vi "Lockin API State Machine.vi"() -> ()   [LabVIEW 2019]
uses:
  Instrument.Lockin/Instrument.Lockin.lvclass
  <userlib>/_OpenG.lib/error/error.llb/openg_error.lvlib
  <userlib>/_OpenG.lib/error/error.llb/Filter Error Codes (Array)__ogtk.vi
  Instrument.Lockin/Typedefs/API/Lockin.Commands--Enum.ctl
  Instrument.Lockin/Typedefs/Results Type--Enum.ctl
  Instrument.DAQ/Typedefs/AO.Channel.Function--Enum.ctl
  Instrument.DAQ/Instrument.DAQ.lvclass
  Instrument.DAQ/Typedefs/AO.Channel--Cluster.ctl
  Instrument.DAQ/Typedefs/AO.Channel--Cluster--Array.ctl
  Instrument.DAQ/Typedefs/REF.Channel--Cluster.ctl
  Instrument.DAQ/Typedefs/REF.Channel--Cluster--Array.ctl
panel:
  in  "Tab Control":T1(tab)=enum."config"
  out "getResults":dbl[](graph)
  in  "Type":T2
  out "getAO":waveform(dbl)[](graph)
  out "getAI":waveform(dbl)[](graph)
  in  "Reset":bool
  in  "Channels: AO":T3 {"Phase" format="%#_3g"; "Frequency" min=0.0001 max=200000.0 format="%#_6p"; "Offset" format="%#_6p"; "Amplitude" min=0.0 max=10.0 format="%#_6p"}
  in  "Channels: Lockin in":T6=[{"Enable?"=FALSE, "Channel"=13, "Frequency"=0.1, "Phase"=0.0, "TC"=1e-05, "Roll-Off"=1}] {"Roll-Off" min=1; "TC" min=0.0001 format="%#_3p"; "Phase" format="%#_3g"; "Frequency" min=0.0001 max=200000.0 format="%#_6p"; "Channel" min=1}
  in  "Trigger":bool
  out "timeout (ms)":u32=202
  in  "side gate channel":i32=1
  in  "phase":dbl
  in  "cycles (1,2,...)":i32=1 min=1 step=1
  in  "Vmin (start)":dbl=-0.15 format="%#_3p"
  in  "Vmax (end)":dbl=0.7 format="%#_3p"
  in  "dV":dbl=0.0005 format="%#_3p"
  in  "function (ramp)":enum16{"Ramp", "Triangle", "Sine"}(ring)
  out "getResults 2":cluster{"Waveform Graph":dbl[], dbl[]}(graph)
  in  "address":string
  in  "Enum":T8
  in  "Stop":bool
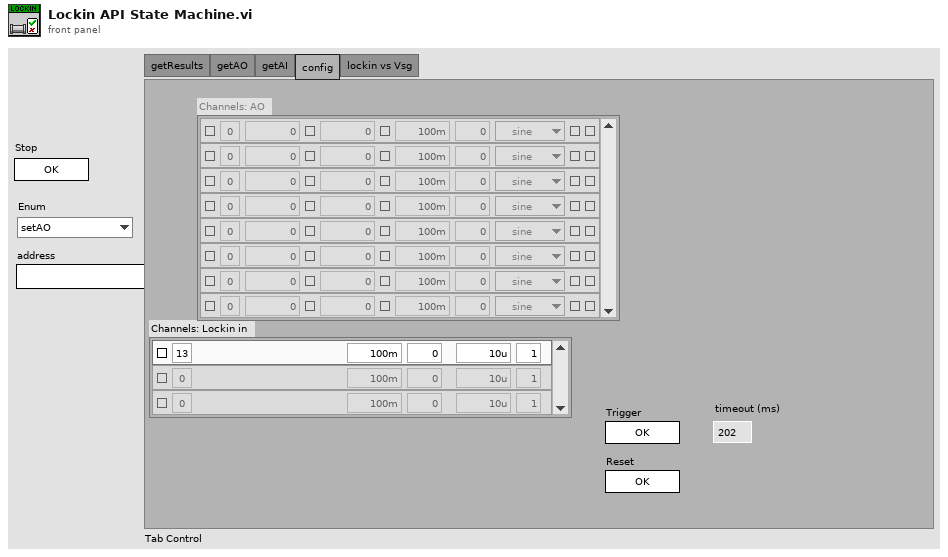
[diagram p1: front panel]
types:
  T1 = enum32{"getResults", "getAO", "getAI", "config", "lockin vs Vsg"}
  T2 = typedef "Instrument.Lockin.lvlib/Instrument.Lockin.lvclass/Results Type--Enum.ctl" = enum16{"X", "Y", "R", "Theta", "Mean"}
  T3 = typedef "Instrument.Lockin.lvlib/Instrument.DAQ.lvclass/AO.Channel--Cluster--Array.ctl" = T4[]
  T4 = typedef "Instrument.Lockin.lvlib/Instrument.DAQ.lvclass/AO.Channel--Cluster.ctl" = cluster{"Enable?":bool, "Channel":i32, "Amplitude":dbl, "Offset":dbl, "Frequency":dbl, "Phase":dbl, "Function":T5, "Sweeping?":bool, "Limit AC":bool, "Limit DC?":bool, "Duty Cycle":bool}
  T5 = typedef "Instrument.Lockin.lvlib/Instrument.DAQ.lvclass/AO.Channel.Function--Enum.ctl" = enum16{"sine", "square", "triangle", "saw"}
  T6 = typedef "Instrument.Lockin.lvlib/Instrument.DAQ.lvclass/REF.Channel--Cluster--Array.ctl" = T7[]
  T7 = typedef "Instrument.Lockin.lvlib/Instrument.DAQ.lvclass/REF.Channel--Cluster.ctl" = cluster{"Enable?":bool, "Channel":i32, "Frequency":dbl, "Phase":dbl, "TC":dbl, "Roll-Off":i32}
  T8 = typedef "Instrument.Lockin.lvlib/Instrument.Lockin.lvclass/Lockin.Commands--Enum.ctl" = enum16{"setAO", "setAO_Amplitude", "setAO_DC", "setAO_Frequency", "setAO_Phase", "setAO_Function", "setREF", "setREF_Frequency", "setREF_Phase", "setREF_TC", "setREF_Roll-Off", "setDAQ", "setSampling", "setState", "getState", "getAO", "getAI", "getResults", "getSampling", "getAOconfig", "getREFconfig", "setInputGain", "setOutputGain", "getInputGain", "getOutputGain", "setSamplingFsMode", "getSamplingFsMode", "setSweep", "setSweep_Time", "setSweep_Table", "getStatus", "getSweepResults", "getSweepWaveforms", "logConfiguration", "startLogging", "stopLogging"}
  T9 = enum32{"invalid app kind", "Development System", "Run Time System", "Student Edition", "Embedded LabVIEW", "Evaluation", "Custom"}
  T10 = enum32{"Invalid", "Standard", "Closed", "Hidden", "Minimized", "Maximized"}
  T11 = cluster{"Core":cluster{"Current VI Reference":refnum<vi>, "Close Panel on Exit?":bool}, "Lockin":refnum<class "Instrument.Lockin.lvclass">}
  T12 = cluster{"Current VI Reference":refnum<vi>, "Close Panel on Exit?":bool}
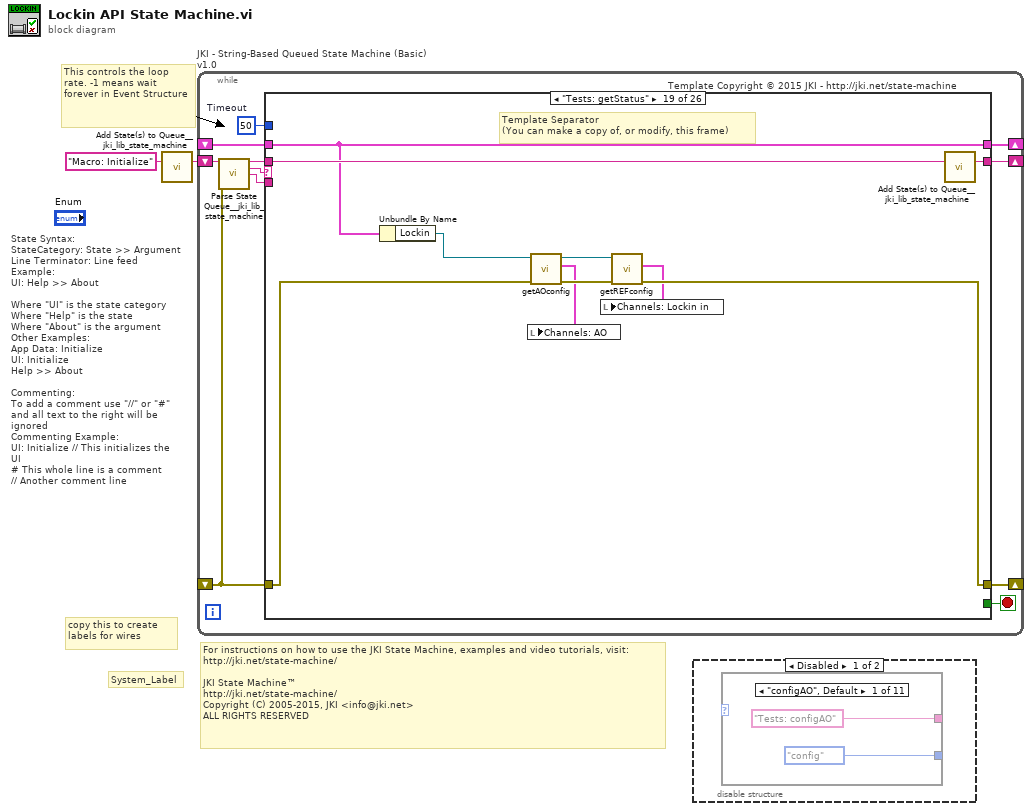
[diagram p0: block diagram]
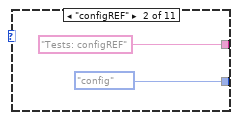
[diagram p2: hidden frame]
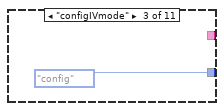
[diagram p3: hidden frame]
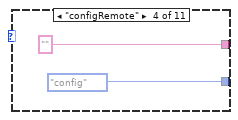
[diagram p4: hidden frame]
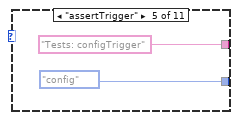
[diagram p5: hidden frame]
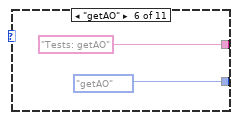
[diagram p6: hidden frame]
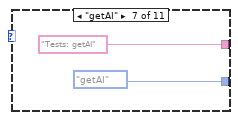
[diagram p7: hidden frame]
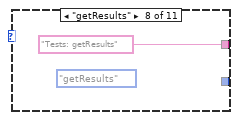
[diagram p8: hidden frame]
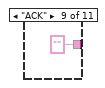
[diagram p9: hidden frame]
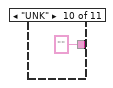
[diagram p10: hidden frame]
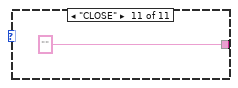
[diagram p11: hidden frame]
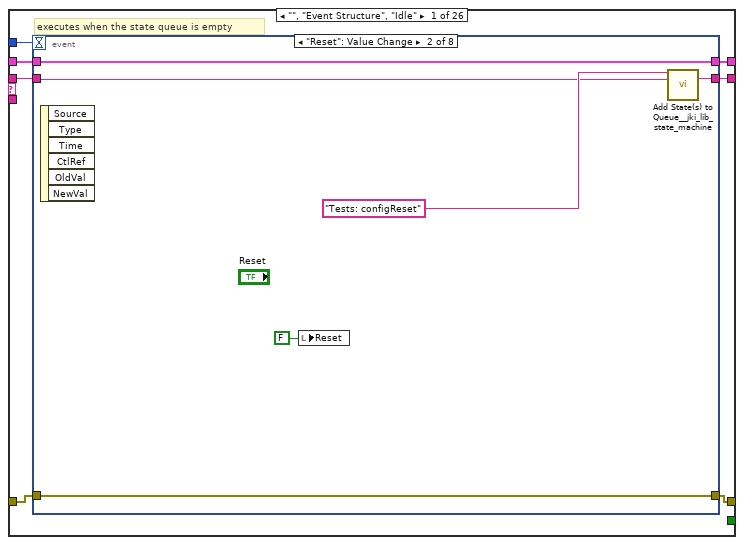
[diagram p13: hidden frame]
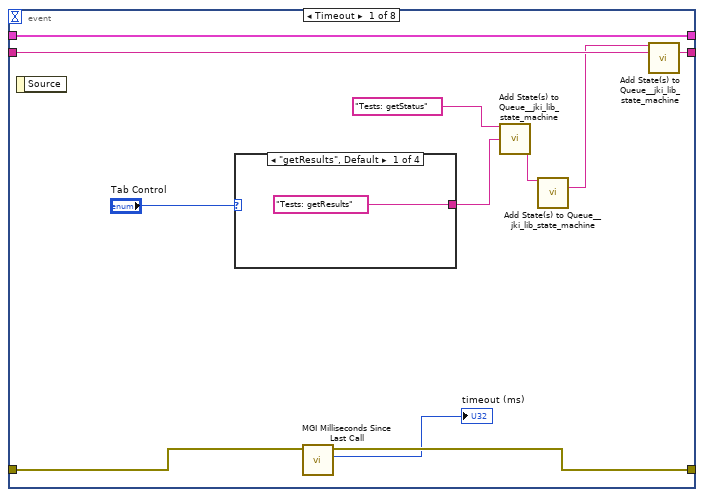
[diagram p14: hidden frame]
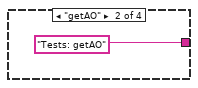
[diagram p15: hidden frame]
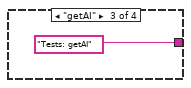
[diagram p16: hidden frame]
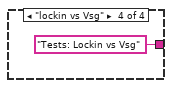
[diagram p17: hidden frame]
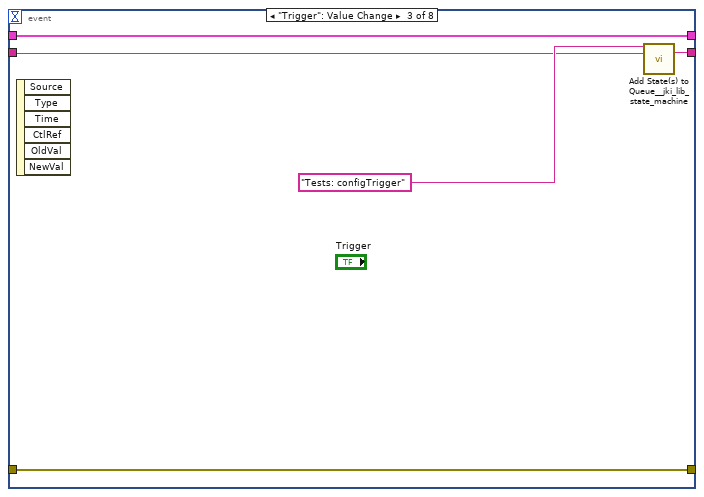
[diagram p18: hidden frame]
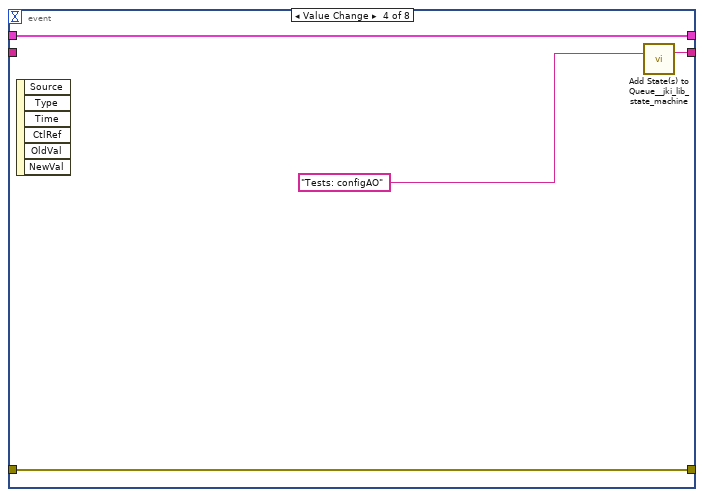
[diagram p19: hidden frame]
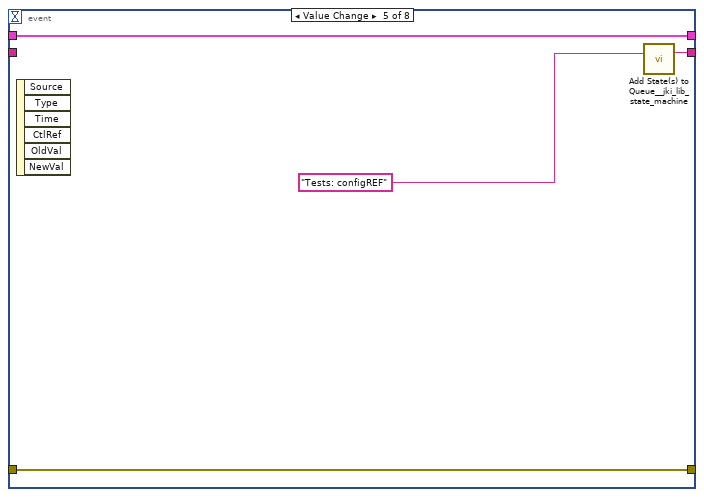
[diagram p20: hidden frame]
diagram:
  # "For instructions on how to use the JKI State Machine, examples and video tutorials, visit:\nhttp://jki.net/state-machine/\n\nJKI State Machine™\nhttp://jki.net/state-machine/\nCopyright (C) 2005-2015, JKI <info@jki.net>\nALL RIGHTS RESERVED"
  # "State Syntax:\nStateCategory: State >> Argument\nLine Terminator: Line feed\nExample:\nUI: Help >> About\n\nWhere \"UI\" is the state category\nWhere \"Help\" is the state\nWhere \"About\" is the argument\nOther Examples:\nApp Data: Initialize\nUI: Initialize\nHelp >> About\n\nCommenting:\nTo add a comment use \"//\" or \"#\" and all text to the right will be ignored\nCommenting Example:\nUI: Initialize // This initializes the UI\n# This whole line is a comment\n// Another comment line"
  # "copy this to create labels for wires"
  # "This controls the loop rate. -1 means wait forever in Event Structure"
  # "System_Label"
  n1 = call <vilib>:"Add State(s) to Queue__jki_lib_state_machine.vi"("State(s) in (\"\")"="Macro: Initialize") -> ("States Out"=w2:string)  [unwired: 14 in]
  n2 = while "JKI - String-Based Queued State Machine (Basic) v1.0" {
    shift-right: [w6] -> _
    shift-left: _ -> [w5]
    shift-right: [w9] -> _
    shift-left: _ -> [w3]
    shift-right: [w8] -> _
    shift-left: w2 -> [w10]
    stop <- w7 stop-if-true
    w4 = 50  # Timeout
    # "Template Copyright © 2015 JKI - http://jki.net/state-machine"
    n3 = call <vilib>:"Parse State Queue__jki_lib_state_machine.vi"("State Queue"=w10, "Error In (no error)"=w3) -> ("Remaining States"=w12:string, "Current State"=w13:string, "Arguments"=w11:string)  [unwired: 11 in]
    n4 = case shown="\"Tests: getStatus\"" w13 {
      selector: w13 -> [_ _ w79 _ _ _ _ _ _ _ _ _ _ _ _ _ _ _ _ _ _ _ _ _ _ _]
      tunnel: w12 -> [w20 w78 w83 w101 w109 w114 w118 w124 w130 w134 w138 w144 w155 w181 w186 w196 w200 w210 w220 w227 w234 w241 w248 w254 w260 w277]
      tunnel: w11 -> [_ _ _ _ _ _ _ _ _ _ _ w139 w149 _ _ _ _ _ _ _ _ _ _ _ _ _]
      tunnel: w5 -> [w18 w75 w81 w92 w106 w112 w115 _ w125 w131 w136 w142 w151 w178 w183 w193 w197 w207 w218 w223 w230 w237 w244 w252 w257 w265]
      tunnel: [w17 w76 w85 w98 errorcluster {"status"=FALSE, "code"=0, "source"=""} ("error out") w111 w116 w121 w126 w132 w135 w140 w152 w179 w184 w194 w198 w201 w215 w224 w231 w238 w245 w250 w256 w275] -> w9
      tunnel: w3 -> [w16 w76 w84 w98 w104 w111 w116 w121 w127 w132 w135 w141 w153 w179 w184 w194 w198 w208 w216 w225 w232 w239 w246 w251 w258 w275]
      tunnel: [w19 w77 w82 w100 w108 w113 w117 w123 w129 w133 w137 w143 w154 w180 w185 w195 w199 w209 w219 w226 w233 w240 w247 w253 w259 w276] -> w8
      tunnel: [_ _ _ _ _ TRUE _ _ _ _ _ _ _ _ _ _ _ _ _ _ _ _ _ _ _ _] -> w7
      tunnel: [w15 w75 w81 w99 w106 w112 w115 w122 w125 w131 w136 w142 w151 w178 w183 w193 w197 w207 w218 w223 w230 w237 w244 w252 w257 w265] -> w6
      tunnel: w4 -> [w14 _ _ _ _ _ _ _ _ _ _ _ _ _ _ _ _ _ _ _ _ _ _ _ _ _]
      frame "", "Event Structure", "Idle" {
        # "executes when the state queue is empty"
        n5 = event shown="[1] \"Reset\": Value Change" {
          selector: _ -> [_ _ _ _ _ _ _ _]
          dyn-events: _ -> [_ _ _ _ _ _ _ _]
          timeout: w14 -> [_ _ _ _ _ _ _ _]
          tunnel: w20 -> [w31 w37 w42 _ _ w62 w68 w74]
          tunnel: [w30 w41 w46 w50 w54 w63 w67 w73] -> w19
          tunnel: w18 -> [w29 w38 w43 w48 w52 w58 w65 w71]
          tunnel: [w22 w39 w44 w49 w53 w55 w66 w72] -> w17
          tunnel: w16 -> [w23 w39 w44 w49 w53 w56 w66 w72]
          tunnel: [w29 w38 w43 w48 w52 w61 w65 w71] -> w15
          event Timeout {
            n6 = event-data() -> ()  [unwired: 1 in, 1 out]
            n7 = case shown="\"getResults\", Default" "Tab Control" {
              tunnel: ["Tests: getResults" "Tests: getAO" "Tests: getAI" "Tests: Lockin vs Vsg"] -> w27
              frame "getResults", Default {
              }
              frame "getAO" {
              }
              frame "getAI" {
              }
              frame "lockin vs Vsg" {
              }
            }
            n8 = call <userlib>:"MGI Milliseconds Since Last Call.vi"("Error In"=w23) -> ("ms"=→"timeout (ms)":u32, "Error Out"=w22:errorcluster)  [unwired: 5 in]
            n9 = call <vilib>:"Add State(s) to Queue__jki_lib_state_machine.vi"("State(s) in Front (\"\")"="Tests: getStatus", "State(s) at Back (\"\")"=w27) -> ("States Out"=w25:string)  [unwired: 13 in]
            n10 = call <vilib>:"Add State(s) to Queue__jki_lib_state_machine.vi"("State(s) in Front (\"\")"=w25) -> ("States Out"=w24:string)  [unwired: 14 in]
            n11 = call <vilib>:"Add State(s) to Queue__jki_lib_state_machine.vi"("State(s) in Front (\"\")"=w24, "State(s) in (\"\")"=w31) -> ("States Out"=w30:string)  [unwired: 13 in]
          }
          event "Reset": Value Change {
            n12 = event-data() -> ()  [unwired: 1 in, 6 out]
            n13 = local write "Reset"(FALSE ("Reset")) -> ()
            n14 = call <vilib>:"Add State(s) to Queue__jki_lib_state_machine.vi"("State(s) in Front (\"\")"="Tests: configReset", "State(s) in (\"\")"=w37) -> ("States Out"=w41:string)  [unwired: 13 in]
          }
          event "Trigger": Value Change {
            n15 = event-data() -> ()  [unwired: 1 in, 6 out]
            n16 = call <vilib>:"Add State(s) to Queue__jki_lib_state_machine.vi"("State(s) in Front (\"\")"="Tests: configTrigger", "State(s) in (\"\")"=w42) -> ("States Out"=w46:string)  [unwired: 13 in]
          }
          event Value Change {
            n17 = event-data() -> ()  [unwired: 1 in, 6 out]
            n18 = call <vilib>:"Add State(s) to Queue__jki_lib_state_machine.vi"("State(s) in (\"\")"="Tests: configAO") -> ("States Out"=w50:string)  [unwired: 14 in]
          }
          event Value Change {
            n19 = event-data() -> ()  [unwired: 1 in, 6 out]
            n20 = call <vilib>:"Add State(s) to Queue__jki_lib_state_machine.vi"("State(s) in (\"\")"="Tests: configREF") -> ("States Out"=w54:string)  [unwired: 14 in]
          }
          event "address": Value Change {
            n21 = event-data() -> ()  [unwired: 1 in, 6 out]
            n22 = Unbundle By Name(w58) -> ("Lockin"=w57:refnum<class "Instrument.Lockin.lvclass">)
            n23 = call-dynamic "Open.vi"("error in (no error)"=w56, "address"="address", "Instrument.Lockin in"=w57) -> ("error out"=w55:errorcluster, "Instrument.Lockin out"=w59:refnum<class "Instrument.Lockin.lvclass">)  [unwired: 7 in]
            n24 = Bundle By Name(cluster=w58, "Lockin"=w59) -> (w61:T11)
            n25 = call <vilib>:"Add State(s) to Queue__jki_lib_state_machine.vi"("State(s) in (\"\")"=w62) -> ("States Out"=w63:string)  [unwired: 14 in]
          }
          event "Stop": Value Change {
            # "Exit Button Value Change (pressed) Event\n(this executes Macro: Exit to terminate the VI)"
            n26 = event-data() -> ()  [unwired: 1 in, 1 out]
            n27 = call <vilib>:"Add State(s) to Queue__jki_lib_state_machine.vi"("State(s) in Front (\"\")"="Macro: Exit", "State(s) in (\"\")"=w68) -> ("States Out"=w67:string)  [unwired: 13 in]
          }
          event Panel Close? {
            # "Discard the event because we'll close the front panel ourselves in Macro: Exit"
            # "Close Panel button (pressed) Event\n(this executes Macro: Exit to terminate the VI)"
            n28 = event-data() -> ()  [unwired: 1 in, 1 out]
            n29 = event-data("Discard?"=TRUE) -> ()  [unwired: 1 in, 1 out]
            n30 = call <vilib>:"Add State(s) to Queue__jki_lib_state_machine.vi"("State(s) in Front (\"\")"="Macro: Exit", "State(s) in (\"\")"=w74) -> ("States Out"=w73:string)  [unwired: 13 in]
          }
        }
      }
      frame "---------- Core ----------" {
        # "Do not put any code in this frame.\n(it is a separator no-op)"
        n31 = call <vilib>:"Add State(s) to Queue__jki_lib_state_machine.vi"("State(s) in (\"\")"=w78) -> ("States Out"=w77:string)  [unwired: 14 in]
      }
      frame Default {
        w88 = 42 items=["No error", "Argument error", "Memory is full", "Out of zone", "End of file", "File already open", "Generic file I/O error", "File not found", "File permission error", "Disk is full", "Duplicate path", "Too many files open", "System feature not enabled", "Resource file not found", "Cannot add resource", "Resource not found", "Image not found", "Image memory error", "Pen does not exist", "Config type invalid", "Config token not found", "Config parse error", "Config memory error", "Bad external code format", "Bad external code offset", "External code not present", "Null window", "Destroy window error", "Null menu", "Print aborted", "Bad print record", "Print driver error", "Windows error during printing", "Memory error during printing", "Print dialog error", "Generic print error", "Invalid device refnum", "Device not found", "Device parameter error", "Device unit error", "Cannot open device", "Device call aborted", "Generic error", "Cancelled by user", "Object ID too low", "Object ID too high", "Object not in heap", "Unknown heap", "Unknown object (invalid DefProc)", "Unknown object (DefProc not in table)", "Message out of range", "Invalid (null) method", "Unknown message", "Manager call not supported", "Bad address", "Network operation in progress", "Network operation timed out", "Connection is busy", "Network attribute not supported", "Network error", "Address in use", "System out of memory", "Connection aborted", "Connection refused", "Not connected", "Already connected", "Connection closed", "Initialization error (interapplication manager)", "Bad occurrence", "Wait on unbound occurrence handler", "Occurrence queue overflow", "Datalog type conflict", "Unused", "Unrecognized type (interapplication manager)", "Memory corrupt", "Failed to make temporary DLL", "Old CIN version", "Drag socket not found", "Failed to load drop-object", "Failed to register OLE object", "Failed to release OLE object", "Format specifier type mismatch", "Unknown format specifier", "Too few format specifiers", "Too many format specifiers", "Scan failed", "Newer CIN version", "Error converting to variant", "Runtime menu error", "Password tampered", "Variant attribute not found", "Incompatible variant data type", "Event data is not available", "Event Store is not present", "Occurrence is not found", "Event Queue is not created", "Event info is not available", "Refnum passed is NULL", "Error retrieving Class GUID", "Error retrieving CoClass GUID", "Error retrieving TypeLib GUID.", "Bad built application magic bytes.", "Specific driver is different from the specific driver associated with the Logical Name.", "There is no session opened to the class driver.", "Max Error", "MAX - Error with config objects", "MAX - Error loading configuration", "MAX - Group not supported"]
        # "Current State"
        # "Do not delete, rename, or modify this frame.\n(this is used to capture unhandled states and typos)"
        # "Handle mistyped state name (developer tool)"
        n32 = Format Into String(format string="Software Exception: Unhandled State \"%s\"." ("message"), error in=w84, w79) -> (resulting string=w87:string, error out=w86:errorcluster)  [unwired: 1 in]
        n33 = call <vilib>:"Error Cluster From Error Code.vi"("show call chain? (False)"=TRUE, "error in (no error)"=w86, "error message (\"\")"=w87, "error code (0)"=w88) -> ("error out"=w85:errorcluster)  [unwired: 5 in]
        n34 = call <vilib>:"Add State(s) to Queue__jki_lib_state_machine.vi"("State(s) in (\"\")"=w83) -> ("States Out"=w82:string)  [unwired: 14 in]
      }
      frame "Initialize Core Data" {
        # "Do not delete, rename, or modify this frame.\n(this is used to determine panel behavior on exit)"
        # "originally closed?"
        # "exe?"
        # "If panel starts closed or is an EXE, then close it when we exit"
        n35 = property class="App"() -> ("App.Kind"=w96:T9)  [unwired: 2 in, 2 out]
        n36 = property class="VI"() -> ("Front Panel.Open"=w97:bool)  [unwired: 2 in, 2 out]
        n37 = control-ref of="Current VI Reference"() -> (w90:refnum<vi>)
        n38 = Not(x=w97) -> (.not. x?=w94:bool)
        n39 = Equal?(x=w96, y=T9."Run Time System" ("Application:Kind")) -> (x = y?=w93:bool)
        n40 = Or(x=w94, y=w93) -> (x .or. y?=w91:bool)
        n41 = Bundle By Name(cluster=w92, "Core.Current VI Reference"=w90, "Core.Close Panel on Exit?"=w91) -> (w99:T11)
        n42 = call <vilib>:"Add State(s) to Queue__jki_lib_state_machine.vi"("State(s) in (\"\")"=w101) -> ("States Out"=w100:string)  [unwired: 14 in]
      }
      frame "Error Handler" {
        # "62,63,66 TCP errors\n74 unflatten error resulting from TCP error"
        # "Unhandled Error -- Display it"
        # "Handle any errors here.\nYou can also output any states to clean-up after errors occur"
        # "Clear error"
        n43 = call-poly <userlib>:"Filter Error Codes__ogtk.vi"("Error In"=w104, "Error Codes to Filter"=i32[] [62, 66, 63, 74]) -> ("Error Out"=w103:errorcluster)  [unwired: 7 in, 2 out]
        n44 = call <vilib>:"General Error Handler.vi"("error in (no error)"=w103) -> ()  [unwired: 10 in, 5 out]
        n45 = call <vilib>:"Add State(s) to Queue__jki_lib_state_machine.vi"("State(s) in Front (\"\")"="/* Post Error States", "State(s) in (\"\")"=w109) -> ("States Out"=w108:string)  [unwired: 13 in]
      }
      frame "Exit" {
        # "Do not put any code in this frame.\n(No errors that occur here will be handled.)"
        n46 = call <vilib>:"Add State(s) to Queue__jki_lib_state_machine.vi"("State(s) in (\"\")"=w114) -> ("States Out"=w113:string)  [unwired: 14 in]
      }
      frame "---------- Data ----------" {
        # "Do not put any code in this frame.\n(It is a separator no-op. You can make a copy of this frame to create a new Data frame)"
        n47 = call <vilib>:"Add State(s) to Queue__jki_lib_state_machine.vi"("State(s) in (\"\")"=w118) -> ("States Out"=w117:string)  [unwired: 14 in]
      }
      frame "Data: Initialize" {
        w119 = refnum<class "Instrument.Lockin.lvclass"> refnum  # Lockin
        w120 = T12 {"Current VI Reference"=refnum, "Close Panel on Exit?"=FALSE}  # Core
        # "do not delete - used by framework"
        # "Expand Bundle to add new data elements to shift register data."
        # "Data names and types of shift register data are defined by this bundle."
        # "Initialize the shift-register data, here.\n(data names are defined by what you wire into the bundle function)"
        n48 = Bundle("Core"=w120, "Lockin"=w119) -> (w122:T11)  [unwired: 1 in]
        n49 = call <vilib>:"Add State(s) to Queue__jki_lib_state_machine.vi"("State(s) in (\"\")"=w124) -> ("States Out"=w123:string)  [unwired: 14 in]
      }
      frame "Data: Cleanup" {
        # "Cleanup any data and references, here.\n(this is called automatically, by the Macro: Exit)"
        n50 = Unbundle By Name(w125) -> ("Core.Current VI Reference"=w128:refnum<vi>)
        n51 = Close Reference(reference=w128, error in (no error)=w127) -> (error out=w126:errorcluster)
        n52 = call <vilib>:"Add State(s) to Queue__jki_lib_state_machine.vi"("State(s) in (\"\")"=w130) -> ("States Out"=w129:string)  [unwired: 14 in]
      }
      frame "---------- UI ----------" {
        # "Do not put any code in this frame.\n(It is a separator no-op. You can make a copy of this frame to create a new UI frame)"
        n53 = call <vilib>:"Add State(s) to Queue__jki_lib_state_machine.vi"("State(s) in (\"\")"=w134) -> ("States Out"=w133:string)  [unwired: 14 in]
      }
      frame "UI: Initialize" {
        # "Initialize the User Interface, here.\n(this is called automatically, by the Macro: Init)"
        n54 = call <vilib>:"Add State(s) to Queue__jki_lib_state_machine.vi"("State(s) in (\"\")"=w138) -> ("States Out"=w137:string)  [unwired: 14 in]
      }
      frame "UI: Cursor Set" {
        # "Argument"
        # "Set and Unset Cursor Busy.\n(Usage: \"UI: Cursor Set >> Busy|Idle\")"
        n55 = case shown="\"Idle\", Default" w139 {
          tunnel: w141 -> [w146 w148]
          tunnel: [w145 w147] -> w140
          frame "Idle", Default {
            n56 = call <vilib>:"Unset Busy.vi"("error in (no error)"=w146) -> ("error out"=w145:errorcluster)  [unwired: 10 in]
          }
          frame "Busy" {
            n57 = call <vilib>:"Set Busy.vi"("error in (no error)"=w148) -> ("error out"=w147:errorcluster)  [unwired: 9 in, 1 out]
          }
        }
        n58 = call <vilib>:"Add State(s) to Queue__jki_lib_state_machine.vi"("State(s) in (\"\")"=w144) -> ("States Out"=w143:string)  [unwired: 14 in]
      }
      frame "UI: Front Panel State" {
        # "Argument"
        # "Set Front Panel Open or Closed\n(Usage: \"UI: Front Panel State >> Open|Close\")"
        n59 = Unbundle By Name(w151) -> ("Core.Current VI Reference"=w150:refnum<vi>)
        n60 = case shown="\"Open\", Default" w149 {
          tunnel: w153 -> [w159 w172]
          tunnel: [w161 w173] -> w152
          tunnel: w150 -> [w160 w170]
          frame "Open", Default {
            n61 = property class="VI"(reference=w160, error in=w159) -> (reference out=w157:refnum<vi>, error out=w158:errorcluster, "Front Panel.Open"=w156:bool)
            n62 = case shown="True" w156 {
              tunnel: [w164 w167] -> w161
              tunnel: w158 -> [w163 w167]
              tunnel: w157 -> [w162 _]
              frame False {
                n63 = invoke class="VI" method="FP.Open"(reference=w162, error in=w163, "Activate"=TRUE, "State"=T10."Standard") -> (error out=w164:errorcluster)  [unwired: 1 in, 4 out]
              }
              frame True {
              }
            }
          }
          frame "Close" {
            n64 = property class="VI"(reference=w170, error in=w172) -> (reference out=w169:refnum<vi>, error out=w171:errorcluster, "Front Panel.Open"=w168:bool)
            n65 = case shown="True" w168 {
              tunnel: [w174 w177] -> w173
              tunnel: w171 -> [w174 w176]
              tunnel: w169 -> [_ w175]
              frame False {
              }
              frame True {
                n66 = invoke class="VI" method="FP.Close"(reference=w175, error in=w176) -> (error out=w177:errorcluster)  [unwired: 1 in, 2 out]
              }
            }
          }
        }
        n67 = call <vilib>:"Add State(s) to Queue__jki_lib_state_machine.vi"("State(s) in (\"\")"=w155) -> ("States Out"=w154:string)  [unwired: 14 in]
      }
      frame "---------- Macro ----------" {
        # "Do not put any code in this frame.\n(It is a separator no-op. You can make a copy of this frame to create a new Macro frame)"
        n68 = call <vilib>:"Add State(s) to Queue__jki_lib_state_machine.vi"("State(s) in (\"\")"=w181) -> ("States Out"=w180:string)  [unwired: 14 in]
      }
      frame "Macro: Initialize" {
        w182 = "Data: Initialize\nInitialize Core Data\nUI: Initialize\nUI: Front Panel State >> Open"  # Data: Initialize Initialize Core Data UI: Initialize UI: Front Panel State >> Open
        # "Initialization Macro\n(This is called once, when the VI starts)"
        n69 = call <vilib>:"Add State(s) to Queue__jki_lib_state_machine.vi"("State(s) in Front (\"\")"=w182, "State(s) in (\"\")"=w186) -> ("States Out"=w185:string)  [unwired: 13 in]
      }
      frame "Macro: Exit" {
        # "Exit Macro\n(This is called once, when the VI exits)"
        n70 = Unbundle By Name(w193) -> ("Core.Close Panel on Exit?"=w192:bool)
        n71 = Select(t="UI: Front Panel State >> Close", s=w192, f="") -> (s? t:f=w189:string)
        n72 = call <vilib>:"Add State(s) to Queue__jki_lib_state_machine.vi"("State(s) in (\"\")"=w189, "State(s) at Back (\"\")"="Data: Cleanup\nExit") -> ("States Out"=w187:string)  [unwired: 13 in]
        n73 = call <vilib>:"Add State(s) to Queue__jki_lib_state_machine.vi"("State(s) in Front (\"\")"=w187, "State(s) in (\"\")"=w196) -> ("States Out"=w195:string)  [unwired: 13 in]
      }
      frame "---------- Tests ----------" {
        # "Template Separator\n(You can make a copy of, or modify, this frame)"
        n74 = call <vilib>:"Add State(s) to Queue__jki_lib_state_machine.vi"("State(s) in (\"\")"=w200) -> ("States Out"=w199:string)  [unwired: 14 in]
      }
      frame "Tests: getResults" {
        n75 = Unbundle By Name(w207) -> ("Lockin"=w206:refnum<class "Instrument.Lockin.lvclass">)
        n76 = call-dynamic "getResults.vi"("error in (no error)"=w208, "Instrument.Lockin in"=w206) -> ("error out"=w202:errorcluster, "Results (Dictionary)"=w205:cluster{"key":string, "value":dbl}[])  [unwired: 6 in, 2 out]
        n77 = call "Parse Results (all).vi"("Type"="Type", "error in (no error)"=w202, "Results (Dictionary)"=w205) -> ("error out"=w201:errorcluster, "Data"=→"getResults":dbl[])  [unwired: 5 in, 2 out]
        n78 = call <vilib>:"Add State(s) to Queue__jki_lib_state_machine.vi"("State(s) in (\"\")"=w210) -> ("States Out"=w209:string)  [unwired: 14 in]
      }
      frame "Tests: getStatus" {
        # "Template Separator\n(You can make a copy of, or modify, this frame)"
        n79 = Unbundle By Name(w218) -> ("Lockin"=w212:refnum<class "Instrument.Lockin.lvclass">)
        n80 = call-dynamic "getAOconfig.vi"("error in (no error)"=w216, "Instrument.Lockin in"=w212) -> ("error out"=w217:errorcluster, "AOconfig"=w214:T3, "Instrument.Lockin out"=w211:refnum<class "Instrument.Lockin.lvclass">)  [unwired: 7 in]
        n81 = local write "Channels: AO"(w214) -> ()
        n82 = call-dynamic "getREFconfig.vi"("error in (no error)"=w217, "Instrument.Lockin in"=w211) -> ("error out"=w215:errorcluster, "REFconfig"=w213:T6)  [unwired: 7 in, 1 out]
        n83 = local write "Channels: Lockin in"(w213) -> ()
        n84 = call <vilib>:"Add State(s) to Queue__jki_lib_state_machine.vi"("State(s) in (\"\")"=w220) -> ("States Out"=w219:string)  [unwired: 14 in]
      }
      frame "Tests: getAI" {
        n85 = Unbundle By Name(w223) -> ("Lockin"=w221:refnum<class "Instrument.Lockin.lvclass">)
        n86 = call-dynamic "getAIwfm.vi"("error in (no error)"=w225, "Instrument.Lockin in"=w221) -> ("error out"=w224:errorcluster, "AI Waveform"=→"getAI":waveform(dbl)[])  [unwired: 7 in, 1 out]
        n87 = call <vilib>:"Add State(s) to Queue__jki_lib_state_machine.vi"("State(s) in (\"\")"=w227) -> ("States Out"=w226:string)  [unwired: 14 in]
      }
      frame "Tests: getAO" {
        n88 = Unbundle By Name(w230) -> ("Lockin"=w228:refnum<class "Instrument.Lockin.lvclass">)
        n89 = call-dynamic "getAOwfm.vi"("error in (no error)"=w232, "Instrument.Lockin in"=w228) -> ("error out"=w231:errorcluster, "AO Waveforrm"=→"getAO":waveform(dbl)[])  [unwired: 7 in, 1 out]
        n90 = call <vilib>:"Add State(s) to Queue__jki_lib_state_machine.vi"("State(s) in (\"\")"=w234) -> ("States Out"=w233:string)  [unwired: 14 in]
      }
      frame "Tests: configAO" {
        n91 = Unbundle By Name(w237) -> ("Lockin"=w235:refnum<class "Instrument.Lockin.lvclass">)
        n92 = call-dynamic "setAO.vi"("error in (no error)"=w239, "Channels: AO"="Channels: AO", "Instrument.Lockin in"=w235) -> ("error out"=w238:errorcluster)  [unwired: 7 in, 1 out]
        n93 = call <vilib>:"Add State(s) to Queue__jki_lib_state_machine.vi"("State(s) in (\"\")"=w241) -> ("States Out"=w240:string)  [unwired: 14 in]
      }
      frame "Tests: configREF" {
        n94 = Unbundle By Name(w244) -> ("Lockin"=w242:refnum<class "Instrument.Lockin.lvclass">)
        n95 = call-dynamic "setREF.vi"("error in (no error)"=w246, "Channels: Lockin in"="Channels: Lockin in", "Instrument.Lockin in"=w242) -> ("error out"=w245:errorcluster)  [unwired: 7 in, 1 out]
        n96 = call <vilib>:"Add State(s) to Queue__jki_lib_state_machine.vi"("State(s) in (\"\")"=w248) -> ("States Out"=w247:string)  [unwired: 14 in]
      }
      frame "Tests: configReset" {
        n97 = Unbundle By Name(w252) -> ("Lockin"=w249:refnum<class "Instrument.Lockin.lvclass">)
        n98 = call-dynamic "resetDAQ.vi"("error in (no error)"=w251, "Instrument.Lockin in"=w249) -> ("error out"=w250:errorcluster)  [unwired: 8 in, 1 out]
        n99 = call <vilib>:"Add State(s) to Queue__jki_lib_state_machine.vi"("State(s) in (\"\")"=w254) -> ("States Out"=w253:string)  [unwired: 14 in]
      }
      frame "Tests: configTrigger" {
        n100 = Unbundle By Name(w257) -> ("Lockin"=w255:refnum<class "Instrument.Lockin.lvclass">)
        n101 = call-dynamic "startDAQ.vi"("error in (no error)"=w258, "Instrument.Lockin in"=w255) -> ("error out"=w256:errorcluster)  [unwired: 8 in, 1 out]
        n102 = call <vilib>:"Add State(s) to Queue__jki_lib_state_machine.vi"("State(s) in (\"\")"=w260) -> ("States Out"=w259:string)  [unwired: 14 in]
      }
      frame "Tests: Lockin vs Vsg" {
        n103 = Unbundle By Name(w265) -> ("Lockin"=w261:refnum<class "Instrument.Lockin.lvclass">)
        n104 = call <userlib>:"Max_Min_conversion.vi"("Min"="Vmin (start)", "Max"="Vmax (end)") -> ("offset"=w268:dbl, "Amplitude"=w267:dbl)  [unwired: 8 in]
        n105 = call <userlib>:"Ramp.vi"("phase"="phase", "function (ramp)"="function (ramp)", "cycles (1,2,...)"="cycles (1,2,...)", "step size"="dV", "offset"=w268, "amplitude"=w267) -> ("Waveform Graph"=w264:dbl[])  [unwired: 3 in, 2 out]
        n106 = for {
          tunnel: w264 -> [w285] mode=indexing
          tunnel: "side gate channel" -> [w284]
          tunnel: [w280] -> w263 mode=indexing
          tunnel: w261 -> [w283]
          n107 = call-dynamic "setAO_DC.vi"("DC (V)"=w285, "AO Channel"=w284, "Instrument.Lockin in"=w283) -> ("error out"=w278:errorcluster, "Instrument.Lockin out"=w279:refnum<class "Instrument.Lockin.lvclass">)  [unwired: 7 in]
          n108 = call-dynamic "getResults.vi"("error in (no error)"=w278, "Instrument.Lockin in"=w279) -> ("error out"=w281:errorcluster, "Results (Dictionary)"=w282:cluster{"key":string, "value":dbl}[])  [unwired: 6 in, 2 out]
          n109 = call "Parse Results (single).vi"("error in (no error)"=w281, "Results (Dictionary)"=w282) -> ("Data"=w280:dbl)  [unwired: 6 in, 3 out]
        }
        n110 = Bundle("Waveform Graph"=w264, w263) -> (→"getResults 2":cluster{"Waveform Graph":dbl[], dbl[]})  [unwired: 1 in]
        n111 = call <vilib>:"Add State(s) to Queue__jki_lib_state_machine.vi"("State(s) in (\"\")"=w277) -> ("States Out"=w276:string)  [unwired: 14 in]
      }
    }
  }
  n112 = disable-structure shown="Disabled" {
    frame Disabled {
      n113 = case shown="\"configAO\", Default" {
        selector: _ -> [_ _ _ _ _ _ _ _ _ _ _]
        tunnel: ["Tests: configAO" "Tests: configREF" w291 "" "Tests: configTrigger" "Tests: getAO" "Tests: getAI" "Tests: getResults" "" "" ""] -> _
        tunnel: [enum32{"getResults", "getAO", "getAI", "config"}."config" ("Tab Control") enum32{"getResults", "getAO", "getAI", "config"}."config" ("Tab Control") enum32{"getResults", "getAO", "getAI", "config"}."config" ("Tab Control") enum32{"getResults", "getAO", "getAI", "config"}."config" ("Tab Control") enum32{"getResults", "getAO", "getAI", "config"}."config" ("Tab Control") enum32{"getResults", "getAO", "getAI", "config"}."getAO" ("Tab Control") enum32{"getResults", "getAO", "getAI", "config"}."getAI" ("Tab Control") _ _ _ _] -> _
        frame "configAO", Default {
        }
        frame "configREF" {
        }
        frame "configIVmode" {
        }
        frame "configRemote" {
        }
        frame "assertTrigger" {
        }
        frame "getAO" {
        }
        frame "getAI" {
        }
        frame "getResults" {
          (unwired) enum32{"getResults", "getAO", "getAI", "config"}."getResults" ("Tab Control")
        }
        frame "ACK" {
        }
        frame "UNK" {
        }
        frame "CLOSE" {
        }
      }
    }
    frame Enabled {
    }
  }
